vi "Sub Check Apply or Not.vi"(8 "error in (no error)":errorcluster, 11 "Main Panel in":refnum<class "Main Panel.lvclass">) -> (0 "error out":errorcluster, 2 "Which Button?":T1(ring), 3 "Main Panel out":refnum<class "Main Panel.lvclass">)   [LabVIEW 2018, in "Main Panel.lvlib" / "Main Panel.lvclass"]
uses:
  Main Panel.lvclass
  Main Panel.lvclass/Main Panel.ctl
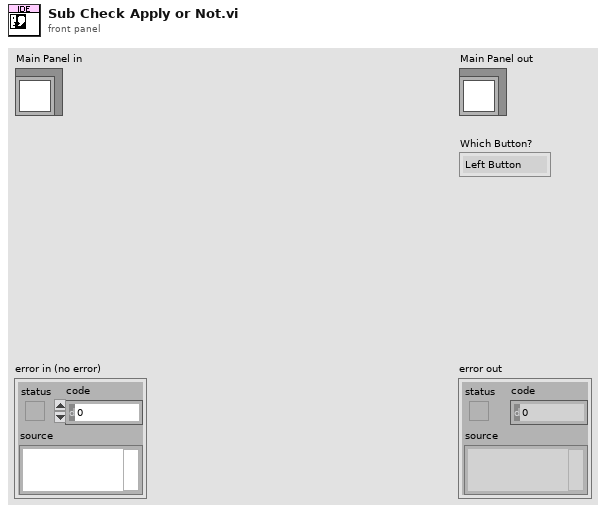
[diagram p1: front panel]
types:
  T1 = enum16{"Left Button", "Center Button", "Right Button", "Window Close"}
  T2 = typedef "Data Parser.lvclass/frame data.ctl" = cluster{"Title":T3, "Basic Data":T4, "Sound":string, "<o> Data":T5, "<bp> Data":T6, "<c> Data":T7, "<w> Data":T8, "<i> Data Array":T9[], "<b> Data Array":T10[]}
  T3 = typedef "Data Parser.lvclass/frame title.ctl" = cluster{"Number":string, "Name":string}
  T4 = typedef "Data Parser.lvclass/frame basic data.ctl" = cluster{"Basic":cluster{"pic":string, "state":string, "wait":string, "next":string}, "Move":cluster{"dvx":string, "dvy":string, "dvz":string}, "Pic Center":cluster{"centerx":string, "centery":string}, "Skill":cluster{"hit_a":string, "hit_d":string, "hit_j":string, "hit_Fa":string, "hit_Ua":string, "hit_Da":string, "hit_Fj":string, "hit_Uj":string, "hit_Dj":string, "hit_ja":string}, "Mp":string}
  T5 = typedef "Data Parser.lvclass/frame o data.ctl" = cluster{"kind":string, "x":string, "y":string, "action":string, "dvx":string, "dvy":string, "dvz":string, "oid":string, "facing":string}
  T6 = typedef "Data Parser.lvclass/frame bp data.ctl" = cluster{"x":string, "y":string}
  T7 = typedef "Data Parser.lvclass/frame c data.ctl" = cluster{"kind":string, "x":string, "y":string, "injury":string, "cover":string, "vaction":string, "aaction":string, "taction":string, "hurtable":string, "decrease":string, "fronthurtact":string, "backhurtact":string, "dircontrol":string, "throwvx":string, "throwvy":string, "throwvz":string, "throwinjury":string}
  T8 = typedef "Data Parser.lvclass/frame w data.ctl" = cluster{"kind":string, "x":string, "y":string, "weaponact":string, "dvx":string, "dvy":string, "dvz":string, "attacking":string, "cover":string}
  T9 = typedef "Data Parser.lvclass/frame i data.ctl" = cluster{"kind":string, "x":string, "y":string, "w":string, "h":string, "dvx":string, "dvy":string, "dvz":string, "fall":string, "arest":string, "vrest":string, "bdefend":string, "injury":string, "zwidth":string, "effect":string, "catchingact":string, "caughtact":string}
  T10 = typedef "Data Parser.lvclass/frame b data.ctl" = cluster{"kind":string, "x":string, "y":string, "w":string, "h":string}
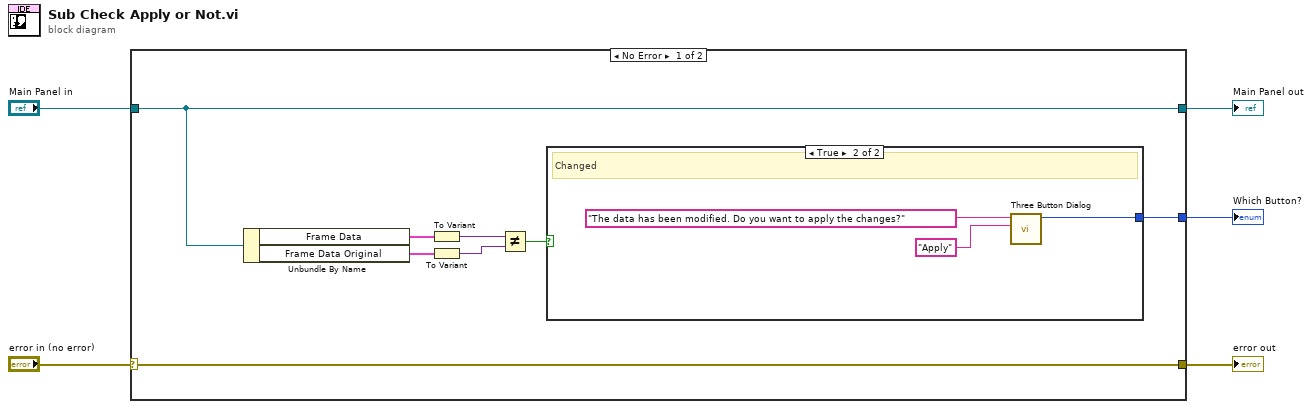
[diagram p0: block diagram]
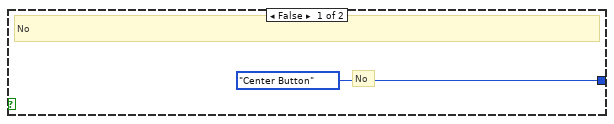
[diagram p2: hidden frame]
diagram:
  n1 = case shown="No Error" "error in (no error)" {
    selector: "error in (no error)" -> [w6 w19]
    tunnel: [w6 w19] -> w4
    tunnel: [w13 w18] -> w2
    tunnel: "Main Panel in" -> [w13 w18]
    tunnel: [w11 _] -> w1
    frame No Error {
      n2 = Unbundle By Name(w13) -> ("Frame Data"=w12:T2, "Frame Data Original"=w7:T2)
      n3 = To Variant(anything=w12) -> (Variant=w9:variant)
      n4 = To Variant(anything=w7) -> (Variant=w10:variant)
      n5 = Not Equal?(x=w9, y=w10) -> (x != y?=w8:bool)
      n6 = case shown="True" w8 {
        tunnel: [T1."Center Button" ("Which Button?") w16] -> w11
        frame False {
          # "No"
          # "No"
        }
        frame True {
          # "Changed"
          n7 = call <vilib>:"Three Button Dialog.vi"("Left Button Text (\"Yes\")"="Apply" ("message"), "message"="The data has been modified. Do you want to apply the changes?") -> ("Which Button?"=w16:T1)  [unwired: 9 in]
        }
      }
    }
    frame Error {
    }
  }
  "error out" <- w4
  "Main Panel out" <- w2
  "Which Button?" <- w1
